vi "Main.vi"(8 "error in":errorcluster, 11 "UserInterface in":refnum<class "UserInterface.lvclass">) -> (0 "error out":errorcluster, 3 "UserInterface out":refnum<class "UserInterface.lvclass">)   [LabVIEW 2017, in "UserInterface.lvclass"]
doc: "The Queued Message Handler of a Worker."
uses:
  UserInterface.lvclass
  Initialization Data.ctl
  <vilib>/addons/_Workers/Library/Classes/Worker/Worker.lvclass
  <vilib>/addons/_Workers/Library/Classes/Message/Message.lvclass
  SimulationDaq/SimulationDaq.lvclass
  <vilib>/addons/_Workers/Library/Classes/Message/Enqueue Message to Self v2.vi
  <vilib>/addons/_Workers/Library/Classes/Message/Enqueue Message to Queue.vi
  <vilib>/addons/_Workers/Library/Classes/Worker/Read ID.vi
  <vilib>/addons/_Workers/Library/Classes/Worker/Read Alias.vi
panel:
  out "ID out":string
  out "Alias out":string
  in  "frequency":dbl=3.3
  in  "amplitude":dbl=1.0
  in  "Button":bool
  out "Waveform Graph":waveform(dbl)(graph)
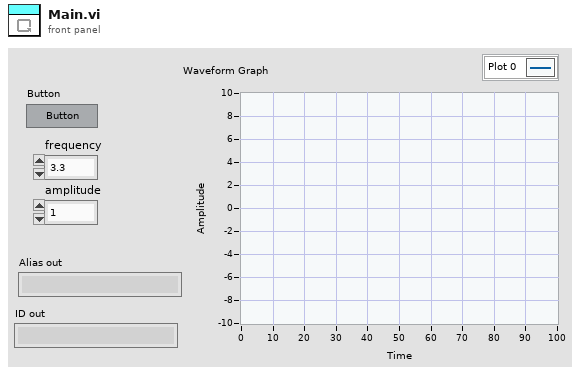
[diagram p1: front panel]
types:
  T1 = typedef "UserInterface.lvclass/Initialization Data.ctl" = cluster{"String":string}
  T2 = cluster{"frequency":dbl, "amplitude":dbl, "sampling info":cluster{"Fs":dbl, "#s":dbl}}
  T3 = typedef "Workers.lvlib/Case Label.ctl" = string
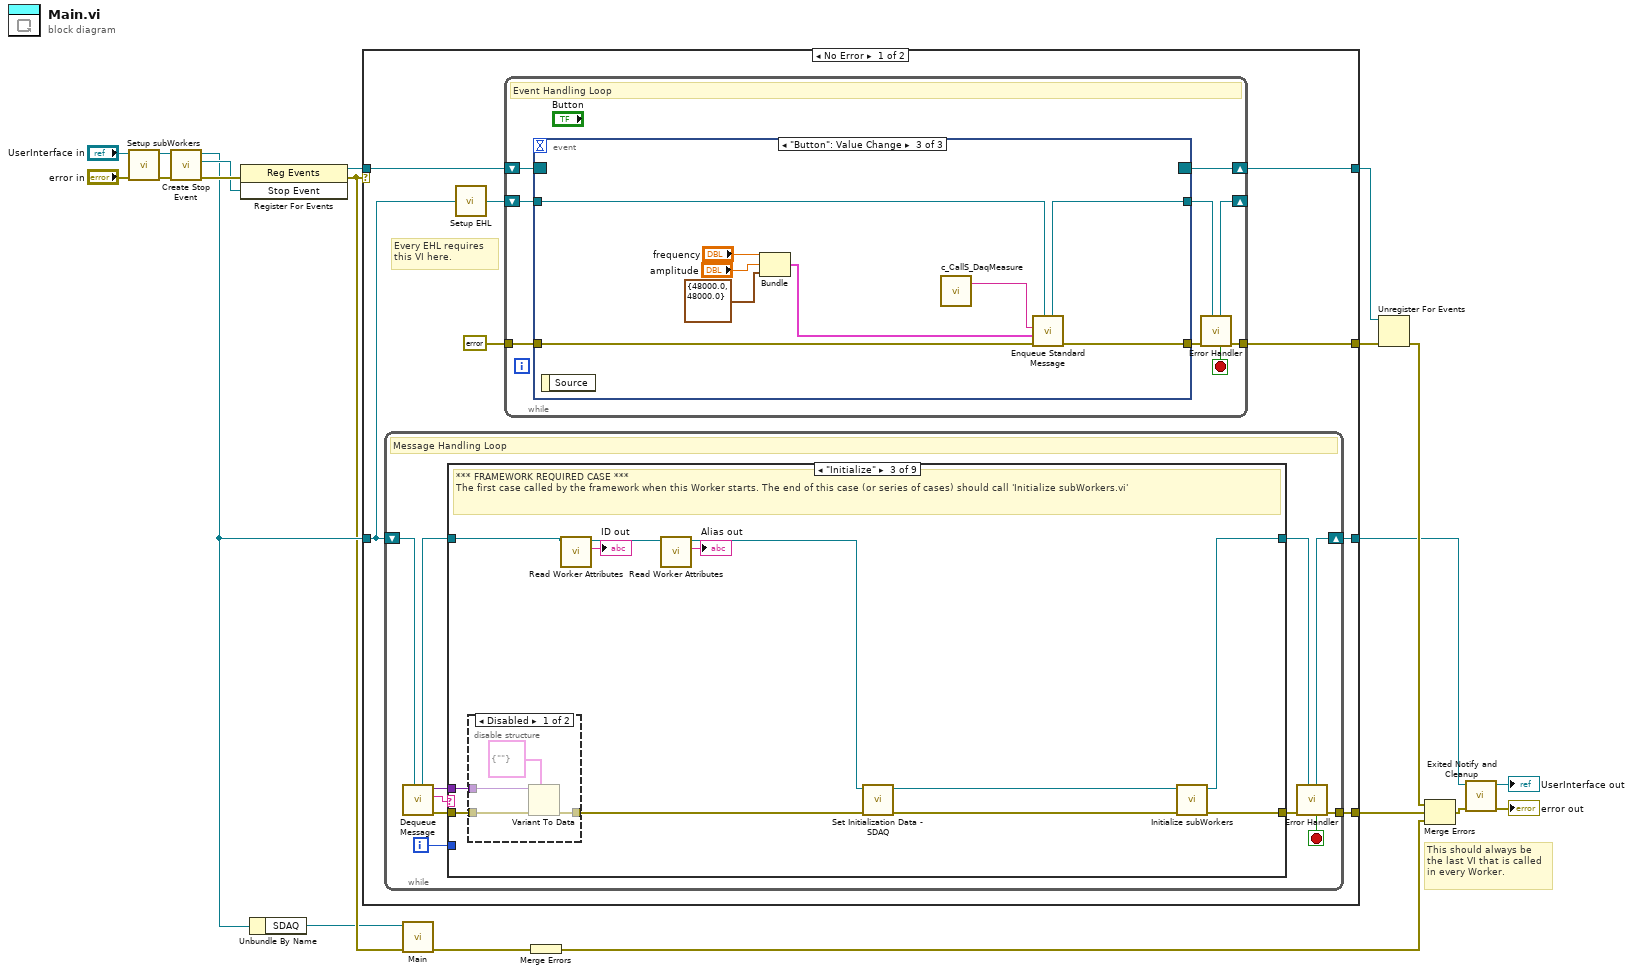
[diagram p0: block diagram]
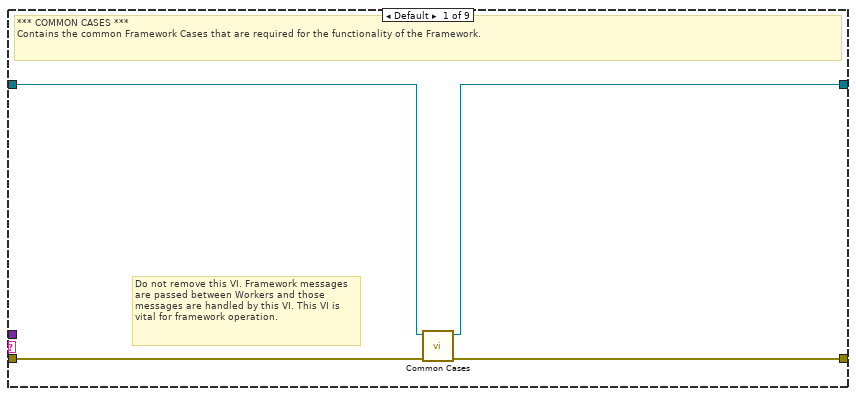
[diagram p2: hidden frame]
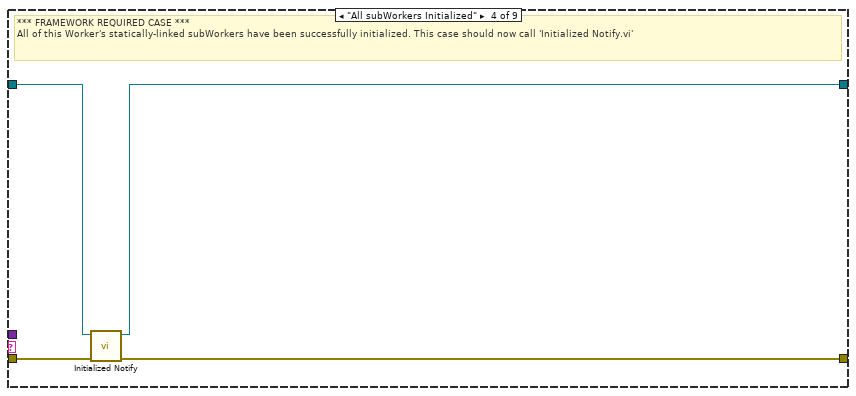
[diagram p5: hidden frame]
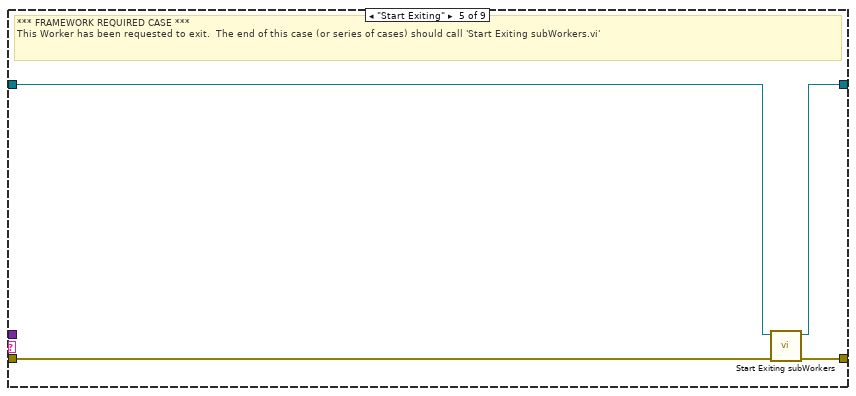
[diagram p6: hidden frame]
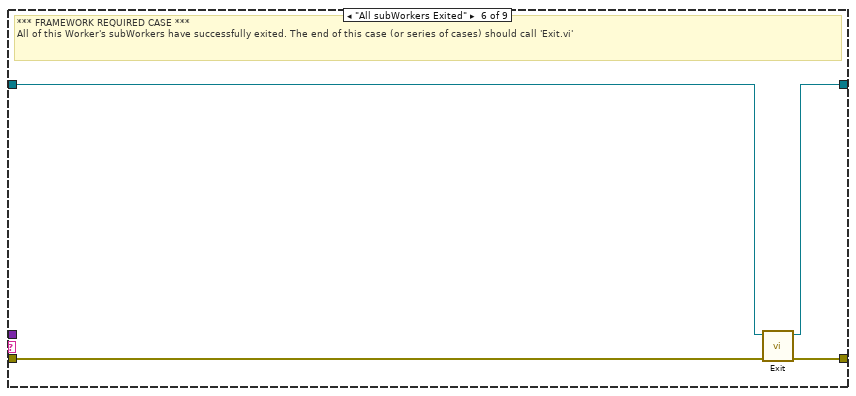
[diagram p7: hidden frame]
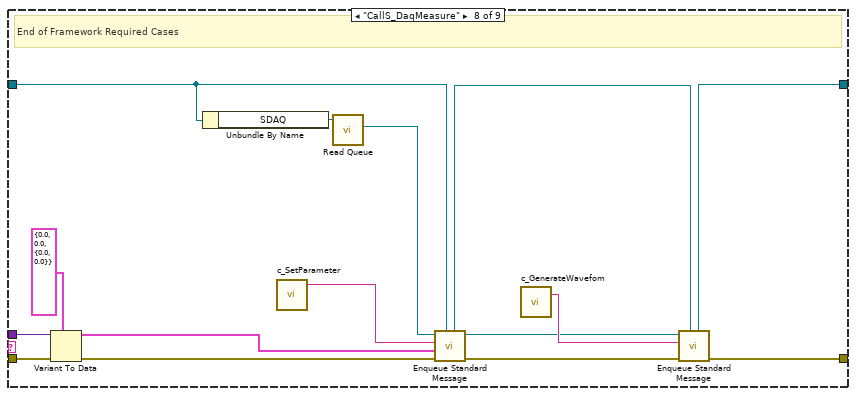
[diagram p9: hidden frame]
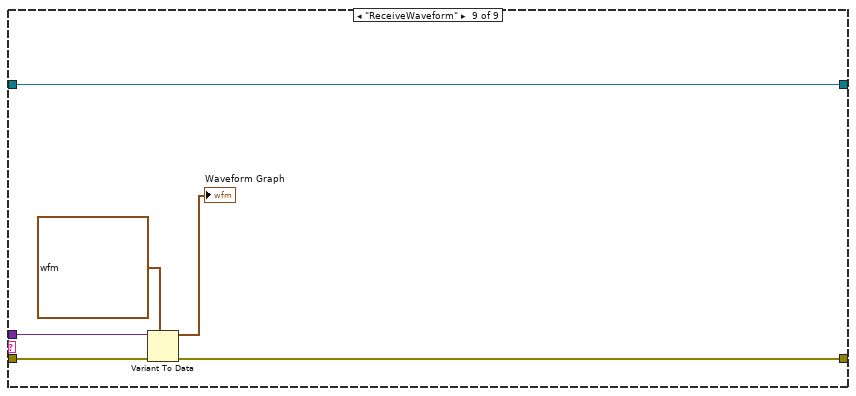
[diagram p10: hidden frame]
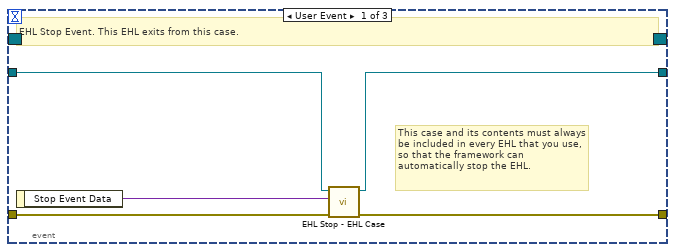
[diagram p11: hidden frame]
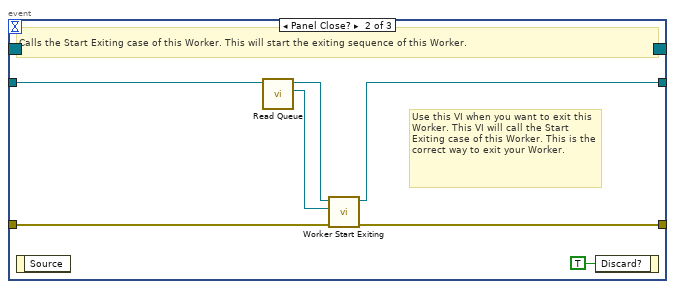
[diagram p12: hidden frame]
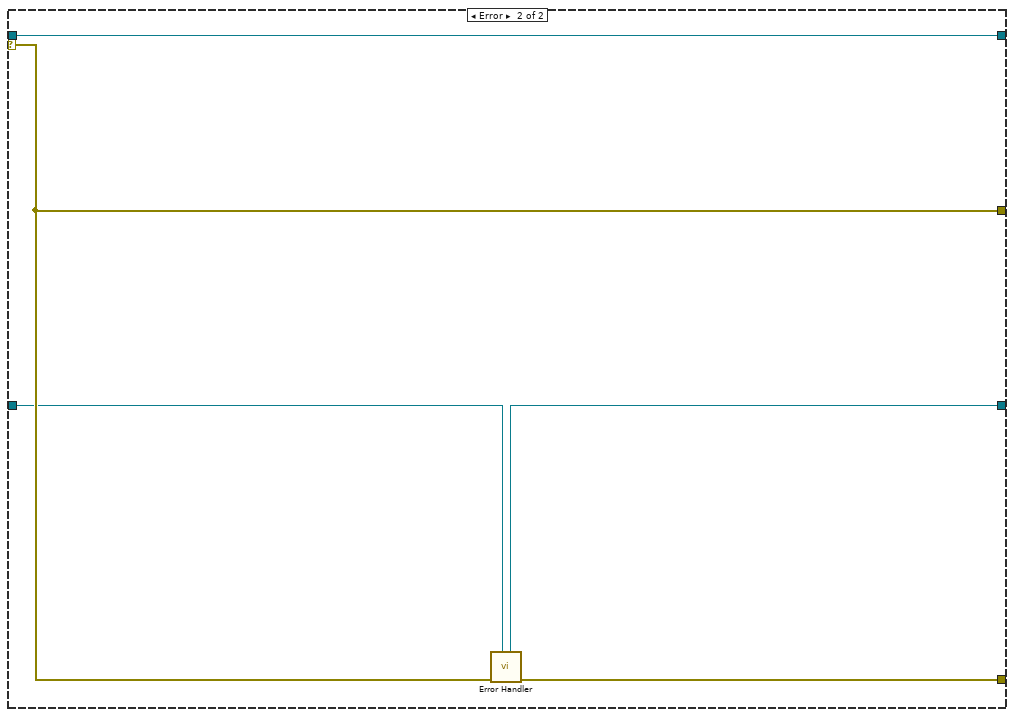
[diagram p13: hidden frame]
diagram:
  # "This should always be the last VI that is called in every Worker."
  n1 = call "Setup subWorkers.vi"("error in"="error in", "UserInterface in"="UserInterface in") -> ("error out"=w6:errorcluster, "UserInterface out"=w4:refnum<class "UserInterface.lvclass">)  [unwired: 8 in]
  n2 = call-dynamic "Create Stop Event.vi"("error in"=w6, "Worker"=w4) -> ("error out"=w15:errorcluster, "Stop Event"=w12:refnum<user-event>, "Worker out"=w9:refnum<class "UserInterface.lvclass">)  [unwired: 7 in]
  n3 = register-events(error in=w15, w12) -> (reference out=w14:refnum<event-registration>, error out=w7:errorcluster)  [unwired: 1 in]
  n4 = Unbundle By Name(w9) -> ("SDAQ"=w1:refnum<class "SimulationDaq.lvclass">)
  n5 = case shown="No Error" w7 {
    tunnel: w9 -> [w23 w129]
    tunnel: [w21 w130] -> w13
    tunnel: w14 -> [w28 w131]
    tunnel: [w25 w132] -> w19
    tunnel: [w27 w131] -> w18
    tunnel: [w22 w128] -> w16
    selector: w7 -> [_ w132]
    frame No Error {
      # "Every EHL requires\nthis VI here."
      n6 = while {
        shift-right: [w37] -> w22
        shift-left: w23 -> [w39]
        tunnel: [w38] -> w21
        i -> [w29]
        stop <- w30 stop-if-true
        # "Message Handling Loop"
        n7 = call-dynamic "Dequeue Message.vi"("Worker"=w39) -> ("error out"=w36:errorcluster, "Case out"=w31:string, "Data out"=w32:variant, "Worker out"=w34:refnum<class "UserInterface.lvclass">)  [unwired: 6 in, 1 out]
        n8 = case "Worker MHL Case Structure (DO NOT CHANGE LABEL NAME)" shown="\"Initialize\"" w31 {
          tunnel: w36 -> [w43 w44 w55 w64 w67 w74 w75 w91 w97]
          tunnel: [w42 w44 w57 w63 w70 w73 w75 w90 w95] -> w35
          tunnel: w34 -> [w41 w45 w49 w66 w68 w72 w76 w81 w96]
          tunnel: [w40 w45 w56 w65 w69 w71 w76 w89 w96] -> w33
          tunnel: w32 -> [_ _ w53 _ _ _ _ w85 w94]
          tunnel: w29 -> [_ _ _ _ _ _ _ _ _]
          frame Default {
            # "Do not remove this VI. Framework messages are passed between Workers and those messages are handled by this VI. This VI is vital for framework operation."
            # "*** COMMON CASES ***\nContains the common Framework Cases that are required for the functionality of the Framework."
            n9 = call-dynamic "Common Cases.vi"("error in"=w43, "Worker in"=w41) -> ("error out"=w42:errorcluster, "Worker out"=w40:refnum<class "UserInterface.lvclass">)  [unwired: 8 in]
          }
          frame "------ FRAMEWORK REQUIRED CASES ------" {
            # "Start of Framework Required Cases"
          }
          frame "Initialize" {
            # "*** FRAMEWORK REQUIRED CASE ***\nThe first case called by the framework when this Worker starts. The end of this case (or series of cases) should call 'Initialize subWorkers.vi'"
            n10 = disable-structure shown="Disabled" {
              disable-tunnel: w55 -> [w61 w62]
              disable-tunnel: [w60 w62] -> w54
              disable-tunnel: w53 -> [w59 _]
              frame Disabled {
                n11 = Variant To Data(error in=w61, type=T1 {"String"=""} ("Initialization Data"), Variant=w59) -> (error out=w60:errorcluster)  [unwired: 1 out]
              }
              frame Enabled {
              }
            }
            n12 = call-poly <vilib>:"Read Worker Attributes.vi"("Worker"=w49) -> ("ID out"=→"ID out":string, "dup Worker out"=w50:refnum<class "UserInterface.lvclass">)  [unwired: 9 in]
            n13 = call-poly <vilib>:"Read Worker Attributes.vi"("Worker"=w50) -> ("Alias out"=→"Alias out":string, "dup Worker out"=w48:refnum<class "UserInterface.lvclass">)  [unwired: 9 in]
            n14 = call "Set Initialization Data - SDAQ.vi"("error in"=w54, "UserInterface in"=w48) -> ("error out"=w52:errorcluster, "UserInterface out"=w51:refnum<class "UserInterface.lvclass">)  [unwired: 8 in]
            n15 = call-dynamic "Initialize subWorkers.vi"("error in"=w52, "Worker"=w51) -> ("error out"=w57:errorcluster, "dup Worker out"=w56:refnum<class "UserInterface.lvclass">)  [unwired: 8 in]
          }
          frame "All subWorkers Initialized" {
            # "*** FRAMEWORK REQUIRED CASE ***\nAll of this Worker's statically-linked subWorkers have been successfully initialized. This case should now call 'Initialized Notify.vi'"
            n16 = call-dynamic "Initialized Notify.vi"("error in"=w64, "Worker"=w66) -> ("error out"=w63:errorcluster, "dup Worker out"=w65:refnum<class "UserInterface.lvclass">)  [unwired: 8 in]
          }
          frame "Start Exiting" {
            # "*** FRAMEWORK REQUIRED CASE ***\nThis Worker has been requested to exit.  The end of this case (or series of cases) should call 'Start Exiting subWorkers.vi'"
            n17 = call-dynamic "Start Exiting subWorkers.vi"("error_in"=w67, "Worker"=w68) -> ("error out"=w70:errorcluster, "dup Worker out"=w69:refnum<class "UserInterface.lvclass">)  [unwired: 8 in]
          }
          frame "All subWorkers Exited" {
            # "*** FRAMEWORK REQUIRED CASE ***\nAll of this Worker's subWorkers have successfully exited. The end of this case (or series of cases) should call 'Exit.vi'"
            n18 = call-dynamic "Exit.vi"("error_in"=w74, "Worker"=w72) -> ("error out"=w73:errorcluster, "dup Worker out"=w71:refnum<class "UserInterface.lvclass">)  [unwired: 8 in]
          }
          frame "-----------------------------------------------" {
            # "End of Framework Required Cases"
          }
          frame "CallS_DaqMeasure" {
            # "End of Framework Required Cases"
            n19 = Variant To Data(error in=w91, type=T2 {"frequency"=0.0, "amplitude"=0.0, "sampling info"={"Fs"=0.0, "#s"=0.0}} ("output cluster"), Variant=w85) -> (data=w77:T2, error out=w86:errorcluster)
            n20 = Unbundle By Name(w81) -> ("SDAQ"=w88:refnum<class "SimulationDaq.lvclass">)
            n21 = call "c_SetParameter.vi"() -> ("Case Label"=w78:T3)  [unwired: 1 in]
            n22 = call <vilib>:"Read Queue.vi"("Worker"=w88) -> ("Message Queue out"=w80:refnum<class "Message Queue.lvclass">)  [unwired: 9 in, 1 out]
            n23 = call-poly <vilib>:"Enqueue Standard Message.vi"("Worker"=w81, "error in"=w86, "Data"=w77, "Case Label"=w78, "Message Queue"=w80) -> ("error out"=w83:errorcluster, "dup Message Queue out"=w79:refnum<class "Message Queue.lvclass">, "dup Worker out"=w82:refnum<class "UserInterface.lvclass">)  [unwired: 4 in]
            n24 = call "c_GenerateWavefom.vi"() -> ("Case Label"=w87:T3)  [unwired: 1 in]
            n25 = call-poly <vilib>:"Enqueue Standard Message.vi"("Worker"=w82, "error in"=w83, "Case Label"=w87, "Message Queue"=w79) -> ("error out"=w90:errorcluster, "dup Worker out"=w89:refnum<class "UserInterface.lvclass">)  [unwired: 5 in, 1 out]
          }
          frame "ReceiveWaveform" {
            n26 = Variant To Data(error in=w97, type=waveform(dbl) {"t0"=timestamp(0 s since 1904-01-01), "dt"=1.0, "Y"=[]} ("Waveform"), Variant=w94) -> (data=→"Waveform Graph":waveform(dbl), error out=w95:errorcluster)
          }
        }
        n27 = call-dynamic "Error Handler.vi"("Worker"=w33, "error_in"=w35) -> ("error out"=w38:errorcluster, "Stop Loop"=w30:bool, "Worker out"=w37:refnum<class "UserInterface.lvclass">)  [unwired: 7 in]
      }
      n28 = call-dynamic "Setup EHL.vi"("Worker"=w23) -> ("Worker out"=w24:refnum<class "UserInterface.lvclass">)  [unwired: 14 in]
      n29 = while "Event Handling Loop" {
        shift-right: [w106] -> w27
        shift-left: w28 -> [w105]
        tunnel: [w101] -> w25
        tunnel: errorcluster {"status"=FALSE, "code"=0, "source"=""} ("error constant") -> [w103]
        shift-right: [w99] -> _
        shift-left: w24 -> [w104]
        stop <- w98 stop-if-true
        # "Event Handling Loop"
        n30 = event shown="[2] \"Button\": Value Change" {
          selector: w105 -> [_ _ _]
          dyn-events: [_ _ _] -> w106
          timeout: _ -> [_ _ _]
          tunnel: [w110 w117 w126] -> w102
          tunnel: w103 -> [w111 w116 w127]
          tunnel: w104 -> [w109 w115 w125]
          tunnel: [w108 w114 w124] -> w100
          event User Event {
            # "This case and its contents must always be included in every EHL that you use, so that the framework can automatically stop the EHL."
            # "EHL Stop Event. This EHL exits from this case."
            n31 = event-data() -> ("Stop Event Data"=w107:variant)  [unwired: 1 in]
            n32 = call <vilib>:"EHL Stop - EHL Case.vi"("error in"=w111, "Stop Event Data"=w107, "Worker"=w109) -> ("error out"=w110:errorcluster, "Worker out"=w108:refnum<class "UserInterface.lvclass">)  [unwired: 7 in]
          }
          event Panel Close? {
            # "Use this VI when you want to exit this Worker. This VI will call the Start Exiting case of this Worker. This is the correct way to exit your Worker."
            # "Calls the Start Exiting case of this Worker. This will start the exiting sequence of this Worker."
            n33 = event-data() -> ()  [unwired: 1 in, 1 out]
            n34 = call <vilib>:"Read Queue.vi"("Worker"=w115) -> ("Message Queue out"=w112:refnum<class "Message Queue.lvclass">, "dup Worker out"=w113:refnum<class "UserInterface.lvclass">)  [unwired: 9 in]
            n35 = call-dynamic "Worker Start Exiting.vi"("error_in"=w116, "Message Queue"=w112, "Worker"=w113) -> ("error out"=w117:errorcluster, "dup Worker out"=w114:refnum<class "UserInterface.lvclass">)  [unwired: 7 in]
            n36 = event-data ("Event Filter Node")("Discard?"=TRUE) -> ()  [unwired: 1 in, 1 out]
          }
          event "Button": Value Change {
            n37 = event-data() -> ()  [unwired: 1 in, 1 out]
            n38 = Bundle("frequency"="frequency", "amplitude"="amplitude", "sampling info"=cluster{"Fs":dbl, "#s":dbl} {"Fs"=48000.0, "#s"=48000.0}) -> (w119:T2)  [unwired: 1 in]
            n39 = call "c_CallS_DaqMeasure.vi"() -> ("Case Label"=w123:T3)  [unwired: 1 in]
            n40 = call-poly <vilib>:"Enqueue Standard Message.vi"("Worker"=w125, "error in"=w127, "Data"=w119, "Case Label"=w123) -> ("error out"=w126:errorcluster, "dup Worker out"=w124:refnum<class "UserInterface.lvclass">)  [unwired: 6 in]
          }
        }
        n41 = call-dynamic "Error Handler.vi"("Worker"=w100, "error_in"=w102) -> ("error out"=w101:errorcluster, "Stop Loop"=w98:bool, "Worker out"=w99:refnum<class "UserInterface.lvclass">)  [unwired: 7 in]
      }
    }
    frame Error {
      n42 = call-dynamic "Error Handler.vi"("Worker"=w129, "error_in"=w132) -> ("error out"=w130:errorcluster, "Worker out"=w128:refnum<class "UserInterface.lvclass">)  [unwired: 7 in, 1 out]
    }
  }
  n43 = call-dynamic "Main.vi"("error in"=w7, "SimulationDaq in"=w1) -> ("error out"=w3:errorcluster)  [unwired: 8 in, 1 out]
  n44 = Merge Errors(w3) -> (w2:errorcluster)
  n45 = Unregister For Events(event registration refnum=w18, error in=w19) -> (error out=w20:errorcluster)
  n46 = Merge Errors(w20, w13, w2) -> (w17:errorcluster)
  n47 = call-dynamic "Exited Notify and Cleanup.vi"("error_in"=w17, "Worker"=w16) -> ("error out"=→"error out":errorcluster, "dup Worker out"=→"UserInterface out":refnum<class "UserInterface.lvclass">)  [unwired: 8 in]
